vi "UT_EField_DAQ_AnalogIO.set channel voltage.vi"(0 "i ref in":refnum<vi>, 3 "Timeout":i32=10000, 5 "error in":errorcluster caption="Fehler (Eingang, kein Fehler)", 9 "channel_index":i32, 11 "voltage":dbl) -> (14 "i ref out":refnum<vi>, 17 "timed out":bool, 19 "error out":errorcluster caption="Fehler (Ausgang)")   [LabVIEW 2014, in "UT_EField_DAQ_AnalogIO.lvlib"]
doc: "Contact: Falk Ziegler, eMail: info@lab-coding.de"
uses:
  UT_EField_DAQ_AnalogIO.lvlib
  CSCore/CSSystem/CoreDefs/CoreDefs.error_type.ctl
  CSCore/CSApplicationBaseClasses/PSChannelBase/PSChannelBase.directionType.ctl
  CSCore/CSApplicationBaseClasses/PSChannelBase/PSChannelBase.serviceType.ctl
  CSlibraries/UtilityLib/UtilityLib.valueStatus.ctl
  <vilib>/DAQmx/write.llb/DAQmx Write (Analog DBL 1Chan 1Samp).vi
  CSCore/CSSystem/CoreLib/CoreLib.lvlib
  CSlibraries/UtilityLib/UtilityLib.lvlib
  CSCore/CSApplicationBaseClasses/DeviceBase/DeviceBase.lvlib
  CSCore/CSApplicationBaseClasses/PSChannelBase/PSChannelBase.lvlib
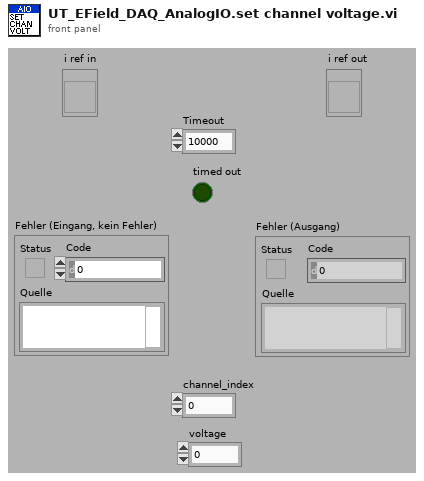
[diagram p1: front panel]
types:
  T1 = typedef "CoreDefs.error_type.ctl" = enum16{"no error", "can't load process", "can't unload process", "process does not exist", "can't install process", "can't remove process", "unknown function", "time out", "can't execute function", "duplicate queue name", "super not found", "caller queue invalid", "can't ping process", "unknown error", "VISA Error", "VISA timeout", "GPIB timeout", "GPIB error", "communication error", "data type mismatch", "can't read data from OPC server", "can't write data to OPC server", "OET error", "function not implemented", "process already exists", "invalid Shared Variable name", "error writing Shared Variable", "error reading Shared Variable", "invalid client name", "corrupt database", "unknown class", "call not authorized", "parameter out of range", "OET timeout: can't get data to modify", "invalid queue name", "requested operation incompatible with current state", "event undefined", "event disabled", "state undefined", "caller is not a friend", "EventBuilder: bad eventID", "EventBuilder: no DAQ devices", "a thread must not stop itself", "UNUSED ELEMENT4", "DiscArchiver: eventData incomplete", "DiscArchiver: eventData does not belong to run", "DiscArchiver: can't open file", "DiscArchiver: can't write to file", "DiscArchiver: available disc space low", "can't acquire semaphore", "error reading data from database", "notifier object is not existing", "can't register process", "can't unregister process", "illegal event type", "object disabled", "object already exists", "can't change state", "Instrument not found", "no connection to remote node", "invalid reference", "N/A", "UNUSED ELEMENT 1", "element not found", "illegal TCP/IP connection detected", "object does not exist", "invalid access ID", "unknown CS system", "invalid privilige", "unsupported data type", "unsupported server type", "IO server already exists", "Shared Variable already exists"}
  T2 = typedef "PSChannelBase.lvlib/PSChannelBase.serviceType.ctl" = enum16{"onOff", "voltage", "current", "tripCurrent", "rampUpSpeed", "rampDownSpeed", "status"}
  T3 = typedef "PSChannelBase.lvlib/PSChannelBase.directionType.ctl" = enum16{"unknown", "update actual value", "update nominal value", "update both"}
  T4 = typedef "UtilityLib.lvlib/UtilityLib.valueStatus.ctl" = enum16{"no info available", "stand by/off", "on", "warning", "alarm/malfunction", "not implemented", "user action required", "important information", "system default", "control default", "indicator default", "button default"}
  T5 = typedef "UT_EField_DAQ_AnalogIO.lvlib/UT_EField_DAQ_AnalogIO.i attribute.ctl" = cluster{"inputs":cluster{"index":i32[], "channel_task":refnum<k21>[], "range":cluster{"min":dbl, "max":dbl}[], "channel_number":i32, "scale_factor":dbl}, "outputs":cluster{"index":i32[], "channel_task":refnum<k21>[], "range":cluster{"min":dbl, "max":dbl}[], "channel_number":i32, "scale_factor":dbl}}
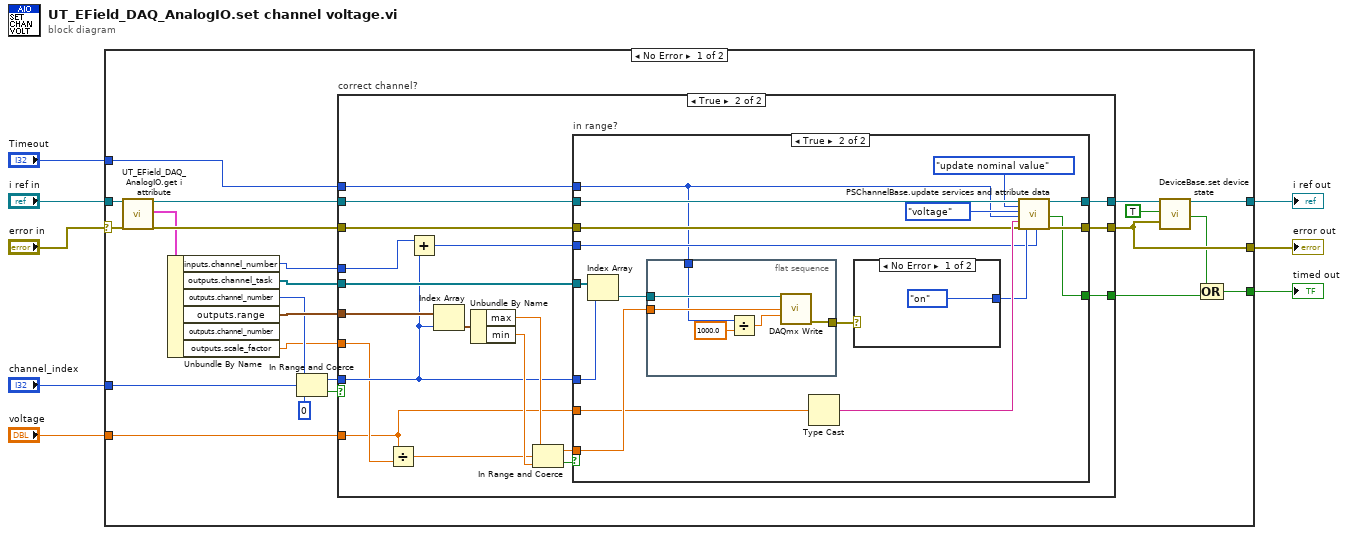
[diagram p0: block diagram]
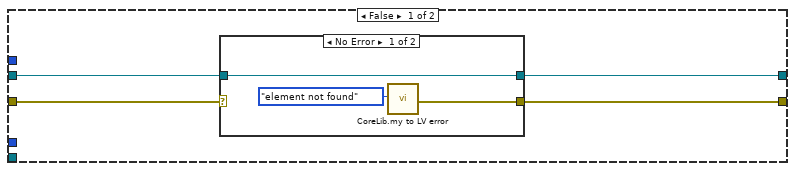
[diagram p2: hidden frame]
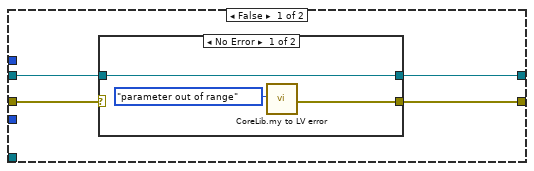
[diagram p4: hidden frame]
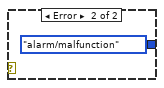
[diagram p6: hidden frame]
diagram:
  n1 = case shown="No Error" "error in" {
    selector: "error in" -> [w30 w94]
    tunnel: "i ref in" -> [w31 w95]
    tunnel: [w23 w95] -> w6
    tunnel: "Timeout" -> [w25 _]
    tunnel: "channel_index" -> [w18 _]
    tunnel: "voltage" -> [w21 _]
    tunnel: [w14 _] -> w2
    tunnel: [w17 w94] -> w1
    frame No Error {
      n2 = call "UT_EField_DAQ_AnalogIO.get i attribute.vi"("i ref in"=w31, "error in (no error)"=w30) -> ("i ref out"=w29:refnum<vi>, "i attribute"=w27:T5, "error out"=w28:errorcluster)  [unwired: 15 in]
      n3 = Unbundle By Name(w27) -> ("inputs.channel_number"=w19:i32, "outputs.channel_task"=w26:refnum<k21>[], "outputs.channel_number"=w10:i32, "outputs.range"=w20:cluster{"min":dbl, "max":dbl}[], "outputs.scale_factor"=w9:dbl)  [unwired: 1 out]
      n4 = In Range and Coerce(upper limit=w10, x=w18, lower limit=0 ("x")) -> (coerced(x)=w13:i32, In Range?=w12:bool)
      n5 = case "correct channel?" shown="True" w12 {
        tunnel: w29 -> [w33 w59]
        tunnel: w28 -> [w34 w55]
        tunnel: w26 -> [_ w48]
        tunnel: w19 -> [_ w44]
        tunnel: w25 -> [_ w58]
        tunnel: [w32 w57] -> w24
        tunnel: [w35 w56] -> w17
        tunnel: [_ w54] -> w15
        tunnel: w21 -> [_ w41]
        tunnel: w20 -> [_ w47]
        tunnel: w13 -> [_ w45]
        tunnel: w9 -> [_ w43]
        frame False {
          n6 = case shown="No Error" w34 {
            selector: w34 -> [_ w40]
            tunnel: [w37 w40] -> w35
            tunnel: w33 -> [w36 w39]
            tunnel: [w36 w39] -> w32
            frame No Error {
              n7 = call "CoreLib.my to LV error.vi"("ErrorTypes"=CoreDefs.error_type."element not found") -> ("myErrorCluster"=w37:errorcluster)  [unwired: 17 in, 1 out]
            }
            frame Error {
            }
          }
        }
        frame True {
          n8 = Divide(x=w41, y=w43) -> (x/y=w42:dbl)
          n9 = Add(x=w44, y=w45) -> (x+y=w46:i32)
          n10 = Index Array(array=w47, index=w45) -> (element=w53:cluster{"min":dbl, "max":dbl})
          n11 = Unbundle By Name(w53) -> ("max"=w51:dbl, "min"=w50:dbl)
          n12 = In Range and Coerce(upper limit=w51, x=w42, lower limit=w50) -> (coerced(x)=w49:dbl, In Range?=w52:bool)
          n13 = case "in range?" shown="True" w52 {
            tunnel: w48 -> [_ w85]
            tunnel: w59 -> [w62 w84]
            tunnel: w58 -> [_ w70]
            tunnel: [w61 w81] -> w57
            tunnel: [w60 w80] -> w56
            tunnel: w55 -> [w63 w79]
            tunnel: [_ w77] -> w54
            tunnel: w49 -> [_ w74]
            tunnel: w45 -> [_ w73]
            tunnel: w46 -> [_ w72]
            tunnel: w41 -> [_ w69]
            frame False {
              n14 = case shown="No Error" w63 {
                selector: w63 -> [_ w68]
                tunnel: [w65 w68] -> w60
                tunnel: w62 -> [w64 w67]
                tunnel: [w64 w67] -> w61
                frame No Error {
                  n15 = call "CoreLib.my to LV error.vi"("ErrorTypes"=CoreDefs.error_type."parameter out of range") -> ("myErrorCluster"=w65:errorcluster)  [unwired: 17 in, 1 out]
                }
                frame Error {
                }
              }
            }
            frame True {
              n16 = Index Array(array=w85, index=w73) -> (element=w83:refnum<k21>)
              n17 = flat-sequence {
                tunnel: w83 -> [w93]
                tunnel: w74 -> [w92]
                tunnel: [w89] -> w71
                tunnel: w70 -> [w88]
                frame #0 {
                  n18 = Divide(x=w88, y=1000.0) -> (x/y=w90:dbl)
                  n19 = call-poly <vilib>:"DAQmx Write.vi"("task/channels in"=w93, "data"=w92, "timeout"=w90) -> ("error out"=w89:errorcluster)  [unwired: 10 in, 2 out]
                }
              }
              n20 = Type Cast(x=w69) -> (*(type *) &x=w82:string)  [unwired: 1 in]
              n21 = case shown="No Error" w71 {
                tunnel: [UtilityLib.valueStatus."on" ("quality") UtilityLib.valueStatus."alarm/malfunction" ("quality")] -> w78
                frame No Error {
                }
                frame Error {
                }
              }
              n22 = call "PSChannelBase.update services and attribute data.vi"("i ref in"=w84, "direction"=PSChannelBase.directionType."update nominal value", "service"=PSChannelBase.serviceType."voltage", "ms timeout (10000)"=w70, "value"=w82, "error in (no error)"=w79, "quality"=w78, "channelNumber"=w72) -> ("i ref out"=w81:refnum<vi>, "timed out"=w77:bool, "error out"=w80:errorcluster)  [unwired: 9 in]
            }
          }
        }
      }
      n23 = call "DeviceBase.set device state.vi"("i ref in"=w24, "implicit"=TRUE, "device error"=w17) -> ("i ref out"=w23:refnum<vi>, "timed out"=w16:bool)  [unwired: 14 in, 1 out]
      n24 = Compound Arithmetic op=OR(w16, w15) -> (w14:bool)
    }
    frame Error {
    }
  }
  "error out" <- w1
  "timed out" <- w2
  "i ref out" <- w6
